vi "Test MQTT-1.5.3-3.vi"(8 "error in (no error)":errorcluster) -> (0 "error out":errorcluster)   [LabVIEW 2013]
uses:
  <vilib>/LabVIEW Open Source Project/MQTT Control Packets/Control Packets/ControlPacket/ControlPacket.lvclass/ControlPacket.ctl
  <vilib>/addons/_JKI Toolkits/Caraya/classes/Test/Test.lvclass
  <vilib>/LabVIEW Open Source Project/MQTT Control Packets/Control Packets/ControlPacket/ControlPacket.lvclass
  <vilib>/LabVIEW Open Source Project/MQTT Control Packets/Control Packets/PUBLISH/PUBLISH.lvclass
  <vilib>/addons/_JKI Toolkits/Caraya/classes/Assert/Assert.lvclass
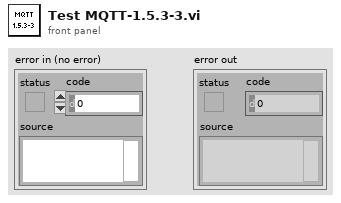
[diagram p1: front panel]
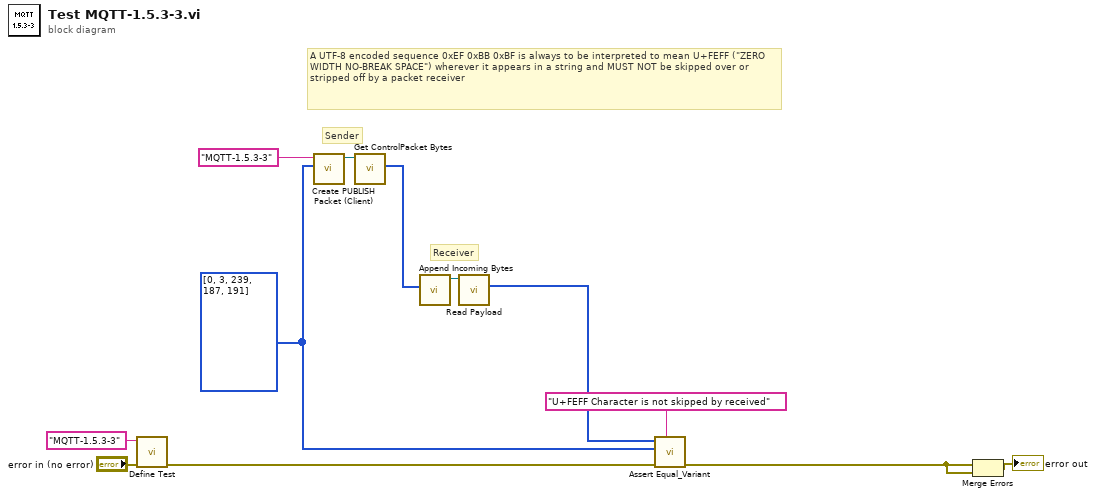
[diagram p0: block diagram]
diagram:
  w1 = u8[] [0, 3, 239, 187, 191] ("Length-Prefixed Field")
  # "Receiver"
  # "Sender"
  # "A UTF-8 encoded sequence 0xEF 0xBB 0xBF is always to be interpreted to mean U+FEFF (\"ZERO WIDTH NO-BREAK SPACE\") wherever it appears in a string and MUST NOT be skipped over or stripped off by a packet receiver"
  n1 = call <vilib>:"Define Test.vi"("error in (no error)"="error in (no error)", "Label (VI Title)"="MQTT-1.5.3-3") -> ("error out"=w8:errorcluster)  [unwired: 9 in]
  n2 = call <vilib>:"Create PUBLISH Packet (Client).vi"("Payload"=w1, "Topic Name"="MQTT-1.5.3-3") -> ("PUBLISH"=w6:refnum<class "PUBLISH.lvclass">)  [unwired: 6 in, 3 out]
  n3 = call <vilib>:"Get ControlPacket Bytes.vi"("ControlPacket"=w6) -> ("Bytes Stream"=w4:u8[])  [unwired: 7 in, 3 out]
  n4 = call <vilib>:"Append Incoming Bytes.vi"("Incoming Packets"=w4) -> ("ControlPacket"=w3:refnum<class "ControlPacket.lvclass">)  [unwired: 7 in, 3 out]
  n5 = call <vilib>:"Read Payload.vi"("ControlPacket in"=w3) -> ("Payload"=w2:u8[])  [unwired: 9 in, 1 out]
  n6 = call <vilib>:"Assert Equal_Variant.vi"("Label"="U+FEFF Character is not skipped by received", "error in (no error)"=w8, "Y"=w1, "X"=w2) -> ("error out"=w7:errorcluster)  [unwired: 7 in]
  n7 = Merge Errors(w7, w7) -> (→"error out":errorcluster)
